vi "Message Send Float.vi"(0 "Value":dbl format="%.2f", 1 "Parameter":string, 2 "Destination":string) -> ()   [LabVIEW 2009]
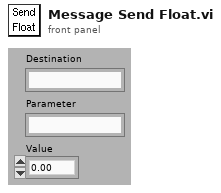
[diagram p1: front panel]
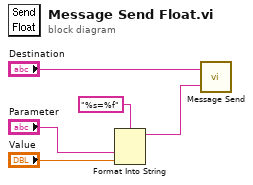
[diagram p0: block diagram]
diagram:
  n1 = Format Into String(format string="%s=%f" ("Format String"), "Parameter", "Value") -> (resulting string=w2:string)  [unwired: 2 in, 1 out]
  n2 = call "Message Send.vi"("Message"=w2, "Destination"="Destination") -> ()
